vi "CRC32.vi"(8 "error in (no error)":errorcluster, 11 "data":u8[](array[numeric])) -> (0 "error out":errorcluster, 3 "crc":u8[](array[numeric]))   [LabVIEW 2023]
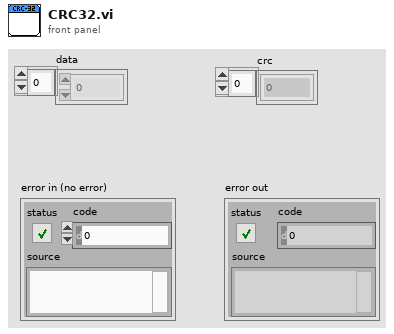
[diagram p1: front panel]
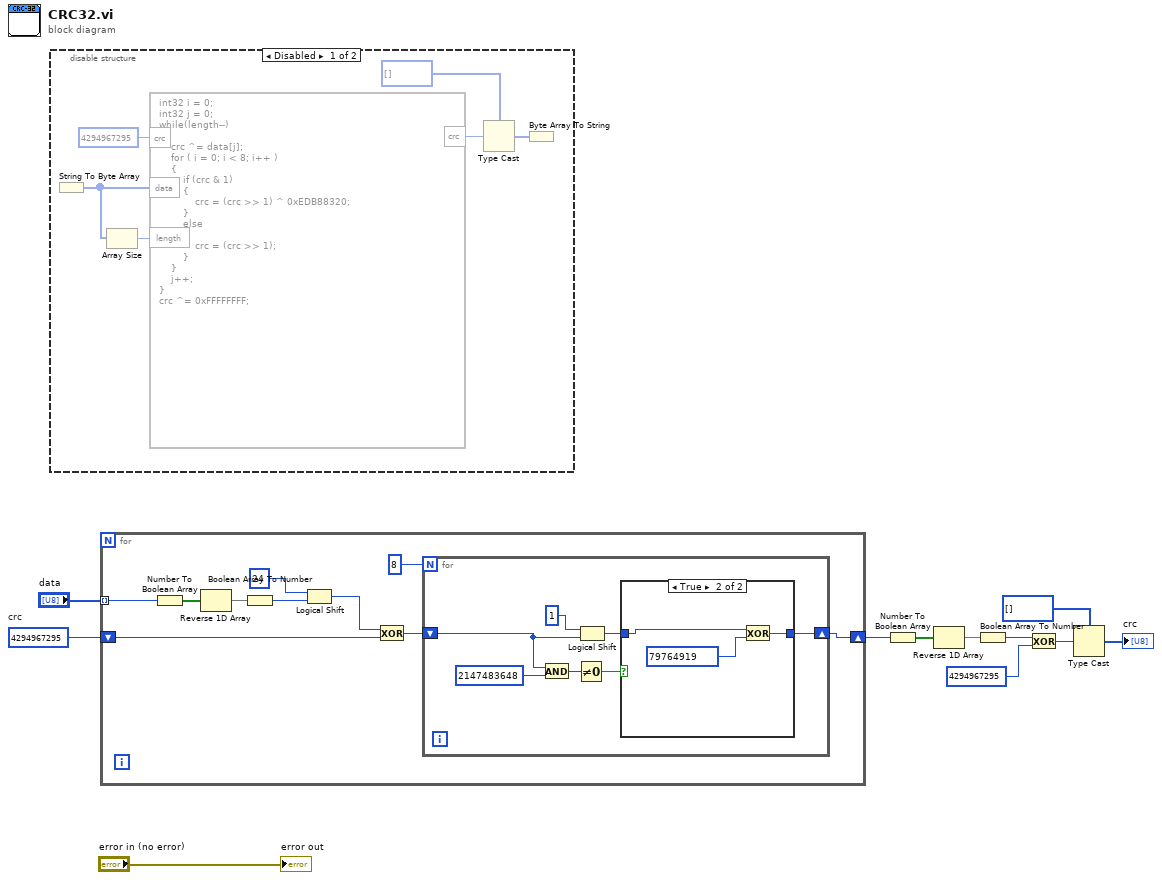
[diagram p0: block diagram]
diagram:
  w6 = u32 4294967295  # crc
  n1 = disable-structure shown="Disabled" {
    frame Disabled {
      n2 = String To Byte Array() -> (unsigned byte array=w17:u8[])  [unwired: 1 in]
      n3 = Array Size(array=w17) -> (size(s)=w16:i32)
      n4 = formula code="int32 i = 0;\nint32 j = 0;\nwhile(length--)\n{\n    crc ^= data[j]; \n    for ( i = 0; i < 8; i++ )\n    {\n        if (crc & 1)\n        {\n            crc = (crc >> 1) ^ 0xEDB88320;\n        }\n        else\n        {\n            crc = (crc >> 1);\n        }\n    }\n    j++;\n}\ncrc ^= 0xFFFFFFFF;"("data"=w17, "length"=w16, "crc"=u32 4294967295) -> ("crc"=w14:u32)
      n5 = Type Cast(type=u8[] [] ("unsigned byte array"), x=w14) -> (*(type *) &x=w12:u8[])
      n6 = Byte Array To String(unsigned byte array=w12) -> ()  [unwired: 1 out]
    }
    frame Enabled {
    }
  }
  n7 = for {
    shift-right: [w24] -> w9
    shift-left: w6 -> [w27]
    tunnel: "data" -> [w21] mode=indexing
    n8 = Number To Boolean Array(number=w21) -> (Boolean array=w23:bool[])
    n9 = Reverse 1D Array(array=w23) -> (reversed array=w22:bool[])
    n10 = Boolean Array To Number(Boolean array=w22) -> (number=w20:u32)
    n11 = Logical Shift(y=i16 24, x=w20) -> (x << y=w18:u32)
    n12 = Exclusive Or(1:w27, 2:w18) -> (0:w25:u32)
    n13 = for {
      N: 8 -> [_]
      shift-right: [w31] -> w24
      shift-left: w25 -> [w30]
      n14 = And(x=w30, y=u32 2147483648 ("x")) -> (x .and. y?=w33:u32)
      n15 = Not Equal To 0?(x=w33) -> (x != 0?=w32:bool)
      n16 = Logical Shift(y=i16 1, x=w30) -> (x << y=w29:u32)
      n17 = case shown="True" w32 {
        tunnel: [w35 w38] -> w31
        tunnel: w29 -> [w35 w37]
        frame False {
        }
        frame True {
          n18 = Exclusive Or(1:u32 79764919, 2:w37) -> (0:w38:u32)
        }
      }
    }
  }
  n19 = Number To Boolean Array(number=w9) -> (Boolean array=w11:bool[])
  n20 = Reverse 1D Array(array=w11) -> (reversed array=w10:bool[])
  n21 = Boolean Array To Number(Boolean array=w10) -> (number=w7:u32)
  n22 = Exclusive Or(1:u32 4294967295, 2:w7) -> (0:w5:u32)
  n23 = Type Cast(type=u8[] [] ("unsigned byte array"), x=w5) -> (*(type *) &x=→"crc":u8[])
  "error out" <- "error in (no error)"
